vi "Interp_2D_Scattered_Data_2_Uniform.vi"(0 "X":dbl[](array[numeric]), 1 "method":i32(ring)=3 items=["nearest", "linear", "cubic", "biharmonic spline "], 2 "Interpolation Factor":i32=1, 5 "Y":dbl[](array[numeric]), 9 "U":dbl[](array[numeric]), 11 "V":dbl[](array[numeric])) -> (3 "IJ Values":i32[](array[numeric]), 4 "Xi":dbl[](array[numeric]), 6 "Yi":dbl[](array[numeric]), 8 "Ui":dbl[](array[numeric]), 10 "Vi":dbl[](array[numeric]), 15 "Convex Hull Check":dbl[](array[numeric]))   [LabVIEW 2011]
uses:
  <vilib>/Math Plots/3D Math Plots/3D Surface/3D Surface XCtrl/3D Surface.xctl
  <vilib>/Math Plots/3D Math Plots/3D Surface/3D Surface Datatype/3D Surface Datatype.lvclass
  <vilib>/Analysis/1siggen.llb/Ramp Pattern by Samples.vi
  <vilib>/gmath/interp.llb/Create Mesh Grid (2D) (x,y arrays).vi
  <vilib>/gmath/interp.llb/Interpolate 2D Scattered (2D).vi
  <vilib>/Math Plots/3D Math Plots/3D Surface/3D Surface Datatype/Public/Plot Helper (Matrix).vi
  <vilib>/gmath/NI_Gmath.lvlib
  <vilib>/Analysis/NI_AALBase.lvlib
  <vilib>/gmath/NI_AAL_Interpolation.lvlib
panel:
  out "3D Surface":refnum<class "3D Plot Datatype.lvclass">[](xcontrol)
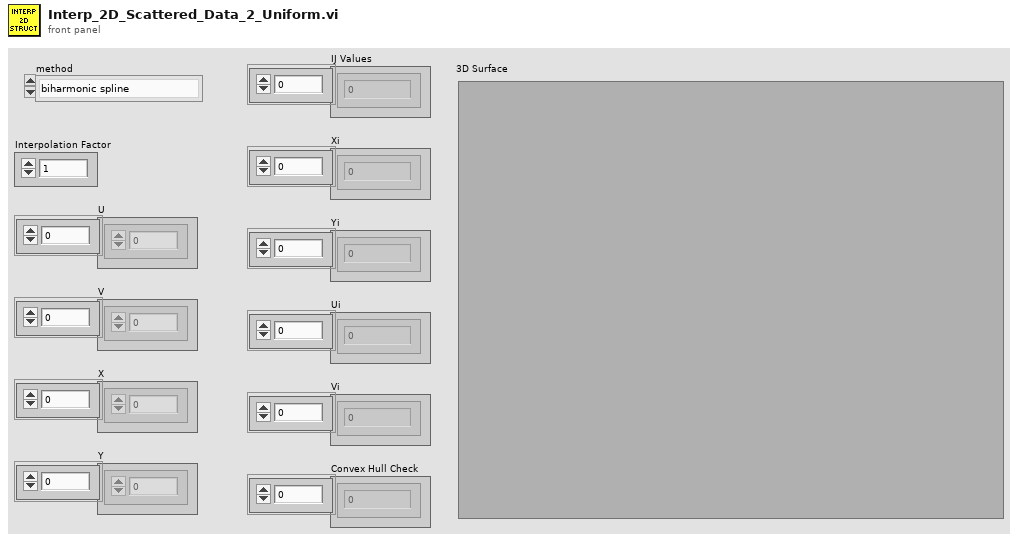
[diagram p1: front panel]
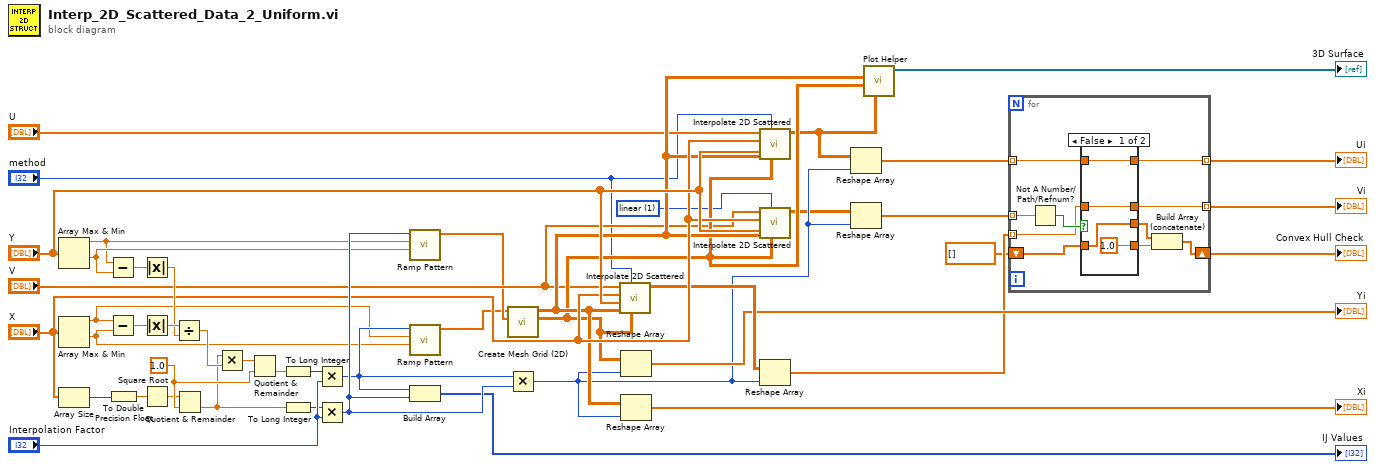
[diagram p0: block diagram]
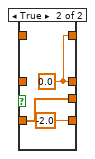
[diagram p2: hidden frame]
diagram:
  w38 = 1.0 ("y")
  w21 = 1 items=["nearest", "linear", "cubic", "biharmonic spline "] ("method")
  n1 = Array Max & Min(array="Y") -> (max value=w24:dbl, min value=w25:dbl)  [unwired: 2 out]
  n2 = Array Max & Min(array="X") -> (max value=w28:dbl, min value=w27:dbl)  [unwired: 2 out]
  n3 = Array Size(array="X") -> (size(s)=w31:i32)
  n4 = Subtract(x=w24, y=w25) -> (x-y=w26:dbl)
  n5 = Subtract(x=w28, y=w27) -> (x-y=w29:dbl)
  n6 = To Double Precision Float(number=w31) -> (double precision float=w32:dbl)
  n7 = Absolute Value(x=w26) -> (abs(x)=w36:dbl)
  n8 = Absolute Value(x=w29) -> (abs(x)=w37:dbl)
  n9 = Square Root(x=w32) -> (sqrt(x)=w33:dbl)
  n10 = Divide(x=w37, y=w36) -> (x/y=w35:dbl)
  n11 = Quotient & Remainder(x=w33, y=w38) -> (floor(x/y)=w34:dbl)  [unwired: 1 out]
  n12 = Multiply(x=w34, y=w35) -> (x*y=w39:dbl)
  n13 = Quotient & Remainder(x=w39, y=w38) -> (floor(x/y)=w40:dbl)  [unwired: 1 out]
  n14 = To Long Integer(number=w40) -> (32bit integer=w42:i32)
  n15 = To Long Integer(number=w34) -> (32bit integer=w44:i32)
  n16 = Multiply(x=w42, y="Interpolation Factor") -> (x*y=w41:i32)
  n17 = Multiply(x=w44, y="Interpolation Factor") -> (x*y=w43:i32)
  n18 = call-poly <vilib>:"Ramp Pattern.vi"("start"=w25, "end"=w24, "samples"=w43) -> ("Ramp Pattern"=w5:dbl[])  [unwired: 7 in, 1 out]
  n19 = call-poly <vilib>:"Ramp Pattern.vi"("start"=w27, "end"=w28, "samples"=w41) -> ("Ramp Pattern"=w4:dbl[])  [unwired: 7 in, 1 out]
  n20 = Build Array(w41, w43) -> (→"IJ Values":i32[])
  n21 = call-poly <vilib>:"Create Mesh Grid (2D).vi"("y domain"=w5, "x domain"=w4) -> ("Y"=w22:dbl[][], "X"=w23:dbl[][])  [unwired: 7 in, 1 out]
  n22 = Multiply(x=w41, y=w43) -> (x*y=w16:i32)
  n23 = call-poly <vilib>:"Interpolate 2D Scattered.vi"("Yi"=w22, "method"="method", "Xi"=w23, "Y"="Y", "X"="X", "Z"="V") -> ("Zi"=w19:dbl[][])  [unwired: 4 in, 1 out]
  n24 = Reshape Array(w22, w16) -> (→"Yi":dbl[])
  n25 = Reshape Array(w23, w16) -> (→"Xi":dbl[])
  n26 = call-poly <vilib>:"Interpolate 2D Scattered.vi"("Yi"=w22, "method"="method", "Xi"=w23, "Y"="Y", "X"="X", "Z"="U") -> ("Zi"=w20:dbl[][])  [unwired: 4 in, 1 out]
  n27 = call-poly <vilib>:"Interpolate 2D Scattered.vi"("Yi"=w22, "method"=w21, "Xi"=w23, "Y"="Y", "X"="X", "Z"="V") -> ("Zi"=w7:dbl[][])  [unwired: 4 in, 1 out]
  n28 = Reshape Array(w19, w16) -> (w13:dbl[])
  n29 = Reshape Array(w20, w16) -> (w12:dbl[])
  n30 = Reshape Array(w7, w16) -> (w8:dbl[])
  n31 = call-poly <vilib>:"Plot Helper.vi"("z matrix"=w20, "y matrix"=w22, "x matrix"=w23) -> ("3D Plot lvclass Array out"=→"3D Surface":refnum<class "3D Plot Datatype.lvclass">[])  [unwired: 3 in, 5 out]
  n32 = for {
    shift-right: [w55] -> w9
    shift-left: dbl[] [] ("output array") -> [w53]
    tunnel: w8 -> [w51] mode=indexing
    tunnel: w12 -> [w50] mode=indexing
    tunnel: w13 -> [w49] mode=indexing
    tunnel: [w48] -> w14 mode=indexing
    tunnel: [w47] -> w15 mode=indexing
    n33 = Not A Number/Path/Refnum?(number/path/refnum=w51) -> (NaN/Path/Refnum?=w56:bool)
    n34 = case shown="False" w56 {
      tunnel: [w60 w63] -> w54
      tunnel: w53 -> [w60 w63]
      tunnel: [1.0 -2.0] -> w52
      tunnel: w50 -> [w58 _]
      tunnel: w49 -> [w57 _]
      tunnel: [w58 w61] -> w48
      tunnel: [w57 w61] -> w47
      frame False {
      }
      frame True {
        w61 = 0.0
      }
    }
    n35 = Build Array (concatenate)(w54, w52) -> (w55:dbl[])
  }
  "Vi" <- w15
  "Ui" <- w14
  "Convex Hull Check" <- w9
